vi "Configure 4Wire Resistance.vi"(0 "VISA resource name":refnum<visa-resource-name>, 1 "Set Aperture or NPLC? (T: Aperture)":bool, 2 "Offset Compensation":bool, 5 "Auto Range? (T: Auto)":bool, 7 "Manual Range":dbl=1000.0, 9 "Aperture Seconds":dbl=0.01616, 11 "error in (no error)":errorcluster, 12 "Enable Dry Circuit":bool, 13 "Detection of Open Leads":bool) -> (4 "VISA resource name out":refnum<visa-resource-name>, 15 "error out":errorcluster)   [LabVIEW 2018, in "Keithley DMM7512.lvlib"]
doc: "This VI configures the 4 wire Resistance."
uses:
  <instrlib>/Keithley DMM7512/Keithley DMM7512.lvlib
panel:
  in  "NPLC":dbl=1.0 min=0.0005 max=15.0 step=1.0
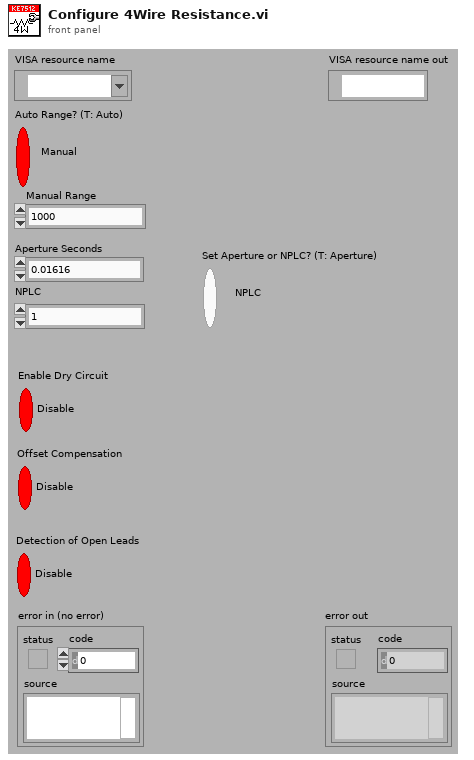
[diagram p1: front panel]
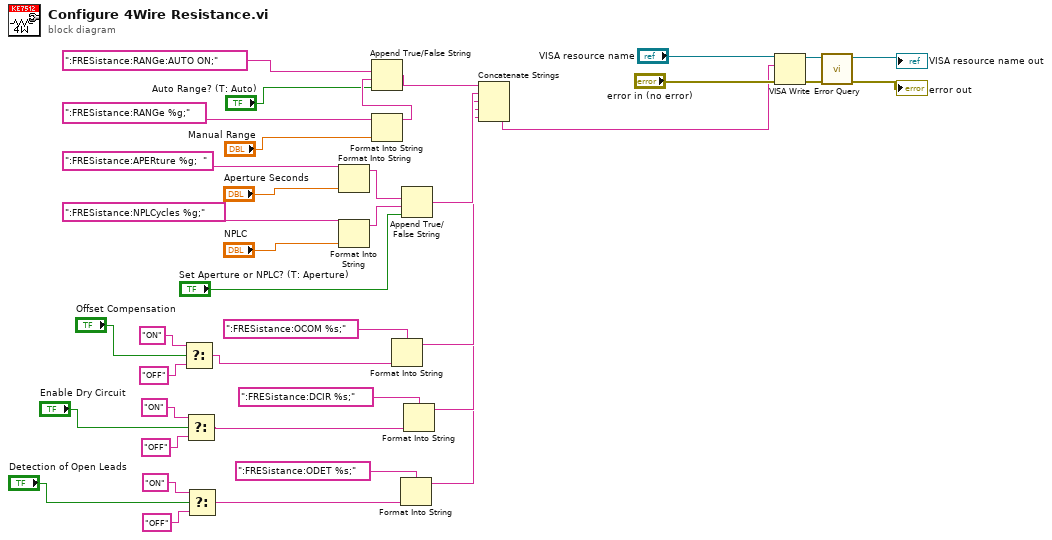
[diagram p0: block diagram]
diagram:
  n1 = Select(t="ON" ("format string"), s="Offset Compensation", f="OFF" ("format string")) -> (s? t:f=w13:string)
  n2 = Select(t="ON" ("format string"), s="Enable Dry Circuit", f="OFF" ("format string")) -> (s? t:f=w9:string)
  n3 = Select(t="ON" ("format string"), s="Detection of Open Leads", f="OFF" ("format string")) -> (s? t:f=w12:string)
  n4 = Format Into String(format string=":FRESistance:APERture %g;  ", "Aperture Seconds") -> (resulting string=w5:string)  [unwired: 2 in, 1 out]
  n5 = Format Into String(format string=":FRESistance:NPLCycles %g;", "NPLC") -> (resulting string=w6:string)  [unwired: 2 in, 1 out]
  n6 = Format Into String(format string=":FRESistance:RANGe %g;", "Manual Range") -> (resulting string=w31:string)  [unwired: 2 in, 1 out]
  n7 = Append True/False String(1:"Auto Range? (T: Auto)", 2:w31, 3:":FRESistance:RANGe:AUTO ON;") -> (0:w28:string)  [unwired: 1 in]
  n8 = Format Into String(format string=":FRESistance:OCOM %s;", w13) -> (resulting string=w3:string)  [unwired: 2 in, 1 out]
  n9 = Format Into String(format string=":FRESistance:ODET %s;", w12) -> (resulting string=w1:string)  [unwired: 2 in, 1 out]
  n10 = Append True/False String(1:"Set Aperture or NPLC? (T: Aperture)", 2:w6, 3:w5) -> (0:w4:string)  [unwired: 1 in]
  n11 = Format Into String(format string=":FRESistance:DCIR %s;", w9) -> (resulting string=w2:string)  [unwired: 2 in, 1 out]
  n12 = Concatenate Strings(w28, w4, w3, w2, w1) -> (w27:string)
  n13 = VISA Write(VISA resource name="VISA resource name", write buffer=w27, error in (no error)="error in (no error)") -> (VISA resource name out=w39:refnum<visa-resource-name>, error out=w38:errorcluster)  [unwired: 1 out]
  n14 = call <instrlib>:"Error Query.vi"("error in (no error)"=w38, "VISA resource name"=w39) -> ("error out"=→"error out":errorcluster, "VISA resource name out"=→"VISA resource name out":refnum<visa-resource-name>)  [unwired: 6 in, 2 out]
